vi "Add.vi"(8 "error in (no error)":errorcluster, 9 "Project":refnum<vi>, 10 "IB_Destination.lvclass":refnum<class "IB_Destination.lvclass">, 11 "IB_Tree_Item_Proj_Container in":refnum<class "IB_Tree_Item_Proj_Container.lvclass">) -> (0 "error out":errorcluster, 1 "updated?":bool, 2 "IB_Source.lvclass":refnum<class "IB_Source.lvclass">, 3 "IB_Tree_Item_Proj_Container out":refnum<class "IB_Tree_Item_Proj_Container.lvclass">)   [LabVIEW 2020, in "IB_Tree_Item_Proj_Container.lvclass"]
uses:
  <vilib>/AppBuilder/IB_Classes/Tree_Item_Proj_Container/IB_Tree_Item_Proj_Container.lvclass
  <vilib>/AppBuilder/IB_Classes/Tree_Item_Proj_Container/IB_Tree_Item_Proj_Container.lvclass/IB_Tree_Item_Proj_Container.ctl
  <vilib>/AppBuilder/IB_Classes/Source/IB_Source.lvclass
  <vilib>/AppBuilder/IB_Classes/Destination/IB_Destination.lvclass
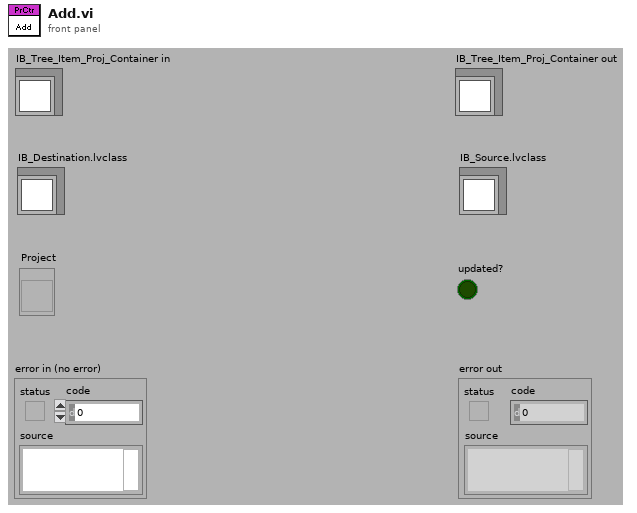
[diagram p1: front panel]
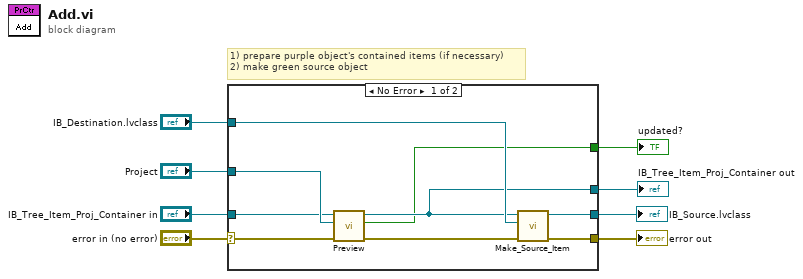
[diagram p0: block diagram]
diagram:
  # "1) prepare purple object's contained items (if necessary)\n2) make green source object"
  n1 = case shown="No Error" "error in (no error)" {
    selector: "error in (no error)" -> [w13 w19]
    tunnel: [w15 w19] -> w7
    tunnel: "IB_Destination.lvclass" -> [w14 _]
    tunnel: "IB_Tree_Item_Proj_Container in" -> [w12 w18]
    tunnel: [w16 _] -> w3
    tunnel: "Project" -> [w17 _]
    tunnel: [w10 w18] -> w2
    tunnel: [w9 _] -> w1
    frame No Error {
      n2 = call-dynamic "Preview.vi"("error in (no error)"=w13, "Project"=w17, "IB_Tree_Item_Proj_Container in"=w12) -> ("error out"=w11:errorcluster, "first preview?"=w9:bool, "IB_Tree_Item_Proj_Container out"=w10:refnum<class "IB_Tree_Item_Proj_Container.lvclass">)  [unwired: 6 in]
      n3 = call-dynamic "Make_Source_Item.vi"("error in (no error)"=w11, "IB_Destination.lvclass"=w14, "IB_Tree_Item_Proj in"=w10) -> ("error out"=w15:errorcluster, "IB_Source.lvclass"=w16:refnum<class "IB_Source.lvclass">)  [unwired: 7 in]
    }
    frame Error {
    }
  }
  "error out" <- w7
  "IB_Source.lvclass" <- w3
  "IB_Tree_Item_Proj_Container out" <- w2
  "updated?" <- w1
